vi "Create Constructor.vi"(8 "error in (no error)":errorcluster, 11 "Mock Class Generator in":refnum<class "Pure Mock Class Generator.lvclass">) -> (0 "error out":errorcluster, 3 "Mock Class Generator":refnum<class "Pure Mock Class Generator.lvclass">)   [LabVIEW 2020, in "Pure Mock Class Generator.lvclass"]
uses:
  Pure Mock Class Generator.lvclass
  Pure Mock Class Generator.lvclass/Pure Mock Class Generator.ctl
  Templates/Template Constructor.vi
  Templates/Templates.lvlib
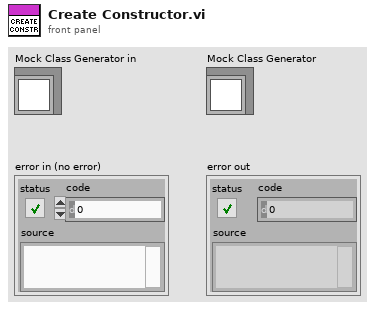
[diagram p1: front panel]
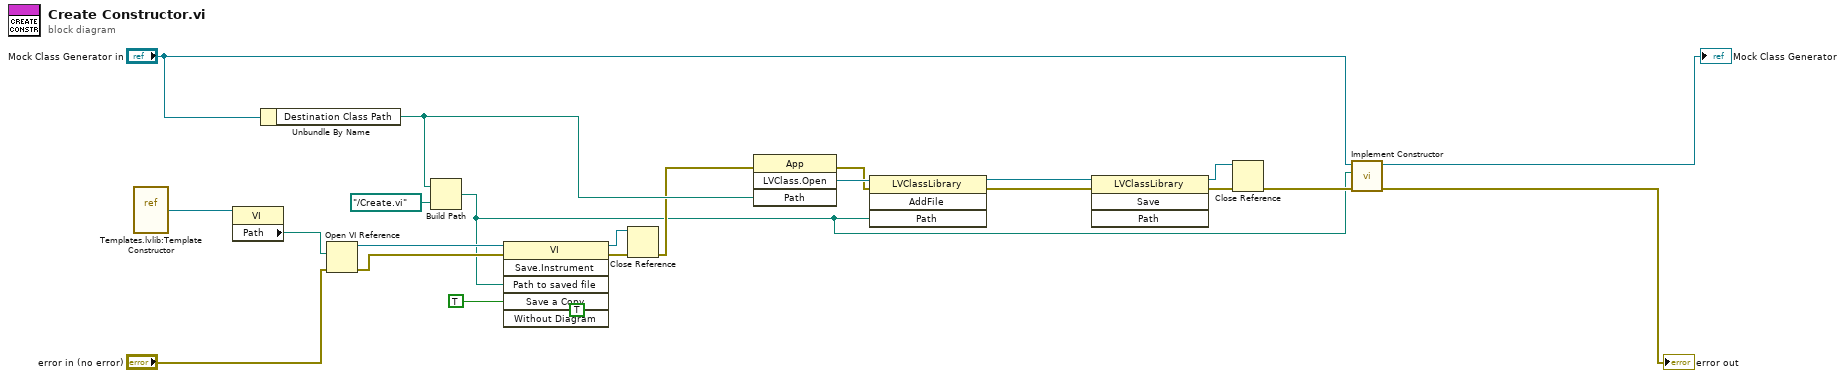
[diagram p0: block diagram]
diagram:
  (unwired) TRUE ("Save a Copy")
  n1 = vi-ref "Templates.lvlib:Template Constructor.vi"() -> (w9:refnum<vi>)
  n2 = property class="VI"(reference=w9) -> ("Path"=w8:path)  [unwired: 1 in, 2 out]
  n3 = Unbundle By Name("Mock Class Generator in") -> ("Destination Class Path"=w19:path)
  n4 = Open VI Reference(vi path=w8, error in (no error)="error in (no error)") -> (vi reference=w10:refnum<vi>, error out=w7:errorcluster)  [unwired: 4 in]
  n5 = Build Path(base path=w19, name or relative path=path "../Create.vi") -> (appended path=w1:path)
  n6 = invoke class="VI" method="Save.Instrument"(reference=w10, error in=w7, "Path to saved file"=w1, "Save a Copy"=TRUE) -> (reference out=w17:refnum<vi>, error out=w20:errorcluster)  [unwired: 2 in, 4 out]
  n7 = Close Reference(reference=w17, error in (no error)=w20) -> (error out=w15:errorcluster)
  n8 = invoke class="App" method="LVClass.Open"(error in=w15, "Path"=w19) -> (error out=w14:errorcluster, "LVClass.Open"=w22:refnum<vi>)  [unwired: 2 in, 2 out]
  n9 = invoke class="LVClassLibrary" method="AddFile"(reference=w22, error in=w14, "Path"=w1) -> (reference out=w13:refnum<vi>, error out=w12:errorcluster)  [unwired: 1 in, 2 out]
  n10 = invoke class="LVClassLibrary" method="Save"(reference=w13, error in=w12) -> (reference out=w5:refnum<vi>, error out=w11:errorcluster)  [unwired: 2 in, 2 out]
  n11 = Close Reference(reference=w5, error in (no error)=w11) -> (error out=w4:errorcluster)
  n12 = call "Implement Constructor.vi"("error in (no error)"=w4, "Constructor Path"=w1, "Mock Class Generator in"="Mock Class Generator in") -> ("error out"=→"error out":errorcluster, "Mock Class Generator"=→"Mock Class Generator":refnum<class "Pure Mock Class Generator.lvclass">)  [unwired: 7 in]
